vi "字模提取.vi"() -> ()   [LabVIEW 2018]
uses:
  46351093-e94a-4c1a-bef4-c87ba8715782.vi
  6c22e504-aebb-492d-a8e3-32474d3b72a3.vi
panel:
  out "字符串 2":string
  out "字符串":string
  out "生成的点阵":bool[][](array[boolean])
  out "new picture 3":picture caption="新图片3"
  out "new picture 2":picture caption="新图片2"
  out "输出灯阵的像素2":i32[](array[numeric])
  in  "布尔 2":bool
  out "new picture":picture caption="新图片"
  out "输出灯阵的像素":i32[](array[numeric])
  out "已删除元素的数组子集":u8[][](array[numeric])
  in  "输入文字":string
  in  "布尔":bool
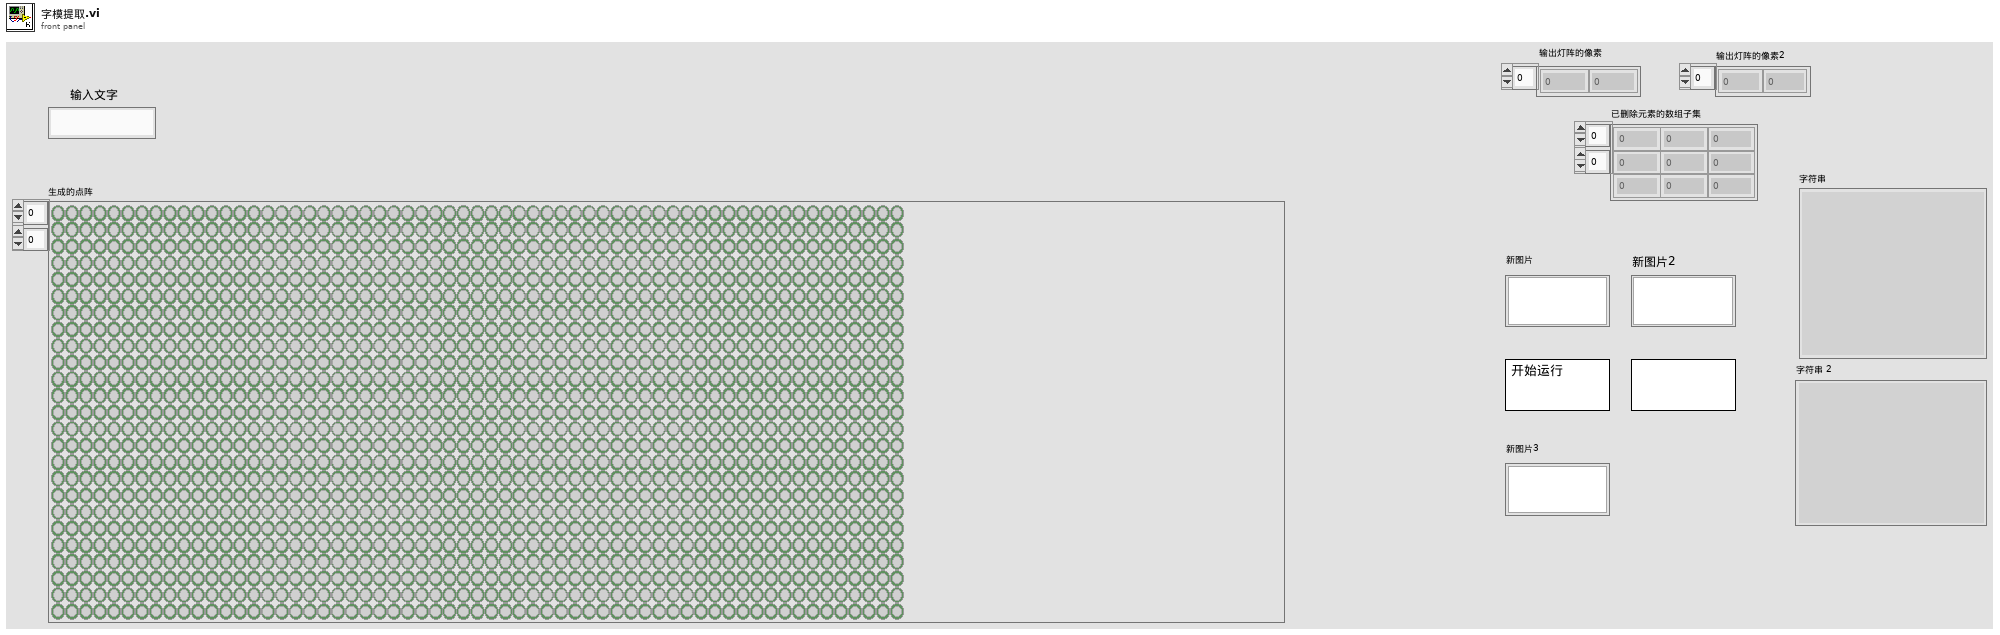
[diagram p1: front panel]
types:
  T1 = typedef "imagedata.ctl" = cluster{"image type":i32, "image depth":i32, "image":u8[], "mask":u8[], "colors":u32[], "Rectangle":cluster{"left":i16, "top":i16, "right":i16, "bottom":i16}}
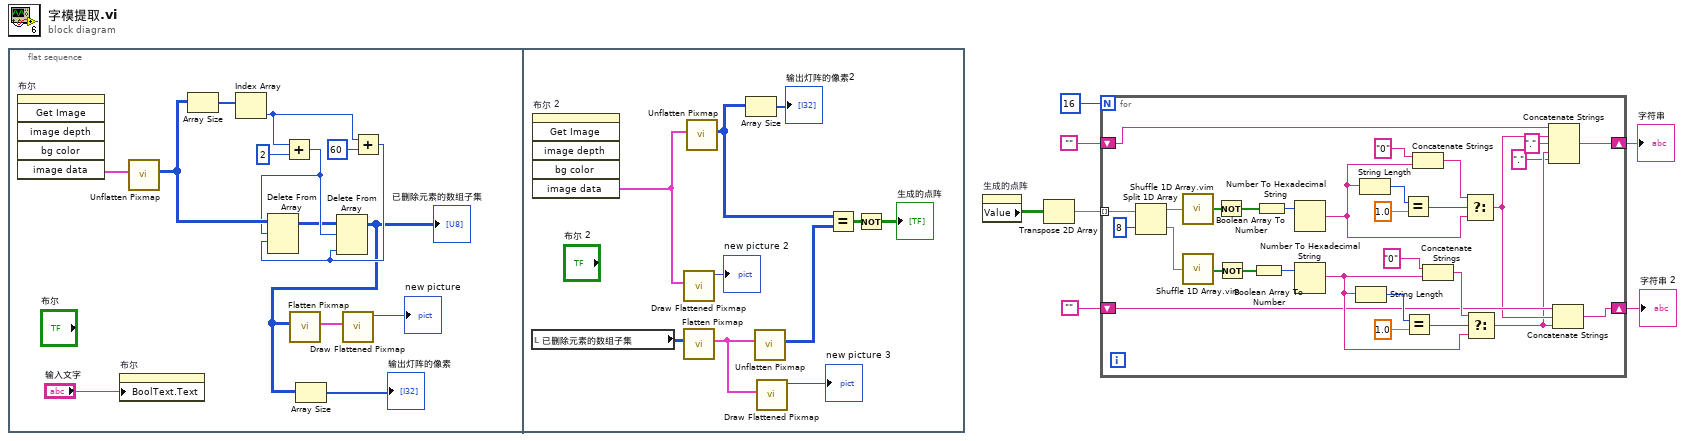
[diagram p0: block diagram]
diagram:
  n1 = flat-sequence {
    frame #0 {
      n2 = invoke on="布尔" class="Bool (严格)" method="Get Image"() -> ("image data"=w20:T1)  [unwired: 6 in, 5 out]
      n3 = property on="布尔" class="Bool (严格)"("BoolText.Text"="输入文字") -> ()  [unwired: 2 in, 2 out]
      n4 = call <vilib>:"Unflatten Pixmap.vi"("image data"=w20) -> ("8-bit pixmap"=w16:u8[][])  [unwired: 4 in, 6 out]
      n5 = Array Size(array=w16) -> (size(s)=w10:i32[])
      n6 = Index Array(array=w10) -> (element=w18:i32)  [unwired: 1 in]
      n7 = Add(x=w18, y=2) -> (x+y=w15:i32)
      n8 = Add(x=w18, y=60) -> (x+y=w11:i32)
      n9 = Delete From Array(array=w16, length=w15, index (row)=w11) -> (array with subset deleted=w9:u8[][])  [unwired: 1 in, 1 out]
      n10 = Delete From Array(array=w9, length=w15, index (col)=w11) -> (array with subset deleted=w8:u8[][])  [unwired: 1 in, 1 out]
      "已删除元素的数组子集" <- w8
      n11 = call <vilib>:"Flatten Pixmap.vi"("8-bit pixmap"=w8) -> ("image data"=w13:T1)  [unwired: 10 in]
      n12 = Array Size(array=w8) -> (size(s)=→"输出灯阵的像素":i32[])
      n13 = call <vilib>:"Draw Flattened Pixmap.vi"("image data"=w13) -> ("new picture"=→"new picture":picture)  [unwired: 8 in]
    }
    frame #1 {
      n14 = local read "已删除元素的数组子集"() -> (w28:u8[][])
      n15 = invoke on="布尔 2" class="Bool (严格)" method="Get Image"() -> ("image data"=w30:T1)  [unwired: 6 in, 5 out]
      n16 = call <vilib>:"Draw Flattened Pixmap.vi"("image data"=w30) -> ("new picture"=→"new picture 2":picture)  [unwired: 8 in]
      n17 = call <vilib>:"Flatten Pixmap.vi"("8-bit pixmap"=w28) -> ("image data"=w27:T1)  [unwired: 10 in]
      n18 = call <vilib>:"Unflatten Pixmap.vi"("image data"=w30) -> ("8-bit pixmap"=w24:u8[][])  [unwired: 4 in, 6 out]
      n19 = Array Size(array=w24) -> (size(s)=→"输出灯阵的像素2":i32[])
      n20 = call <vilib>:"Unflatten Pixmap.vi"("image data"=w27) -> ("8-bit pixmap"=w25:u8[][])  [unwired: 4 in, 6 out]
      n21 = call <vilib>:"Draw Flattened Pixmap.vi"("image data"=w27) -> ("new picture"=→"new picture 3":picture)  [unwired: 8 in]
      n22 = Equal?(x=w24, y=w25) -> (x = y?=w23:bool[][])
      n23 = Not(x=w23) -> (.not. x?=→"生成的点阵":bool[][])
    }
  }
  n24 = property on="生成的点阵" class="Arr (严格)"() -> ("Value"=w5:bool[][])  [unwired: 2 in, 2 out]
  n25 = Transpose 2D Array(2D array=w5) -> (transposed array=w6:bool[][])
  n26 = for {
    N: 16 -> [_]
    shift-right: [w34] -> w3
    shift-left: "" -> [w40]
    shift-right: [w33] -> w1
    shift-left: "" -> [w38]
    tunnel: w6 -> [w61] mode=indexing
    n27 = Split 1D Array(array=w61, index=8 ("索引")) -> (first subarray=w59:bool[], second subarray=w58:bool[])
    n28 = call "Shuffle 1D Array.vim"("array"=w59) -> ("shuffled array"=w57:bool[])  [unwired: 4 in]
    n29 = call "Shuffle 1D Array.vim"("array"=w58) -> ("shuffled array"=w56:bool[])  [unwired: 4 in]
    n30 = Not(x=w57) -> (.not. x?=w54:bool[])
    n31 = Not(x=w56) -> (.not. x?=w53:bool[])
    n32 = Boolean Array To Number(Boolean array=w53) -> (number=w32:u32)
    n33 = Boolean Array To Number(Boolean array=w54) -> (number=w55:u32)
    n34 = Number To Hexadecimal String(2:w55) -> (0:w45:string)  [unwired: 1 in]
    n35 = Number To Hexadecimal String(2:w32) -> (0:w41:string)  [unwired: 1 in]
    n36 = String Length(string=w41) -> (length=w48:i32)
    n37 = String Length(string=w45) -> (length=w47:i32)
    n38 = Equal?(x=w47, y=1.0) -> (x = y?=w52:bool)
    n39 = Equal?(x=w48, y=1.0) -> (x = y?=w49:bool)
    n40 = Concatenate Strings("0" ("字符串"), w45) -> (w46:string)
    n41 = Concatenate Strings("0" ("字符串"), w41) -> (w42:string)
    n42 = Select(t=w46, s=w52, f=w45) -> (s? t:f=w37:string)
    n43 = Select(t=w42, s=w49, f=w41) -> (s? t:f=w36:string)
    n44 = Concatenate Strings(w40, w37, "." ("字符串"), w36, "." ("字符串")) -> (w34:string)
    n45 = Concatenate Strings(w38, w37, w36) -> (w33:string)
  }
  "字符串" <- w3
  "字符串 2" <- w1
